vi "Pulse Pattern.vi"(10 "Selector":T1) -> (2 "Array":u16[](array[numeric]))   [LabVIEW 2026]
uses:
  SideSelector.ctl
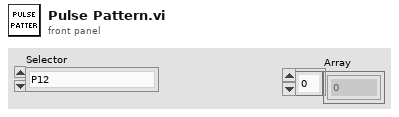
[diagram p1: front panel]
types:
  T1 = typedef "SideSelector.ctl" = enum16{"P12", "P1", "P2"}
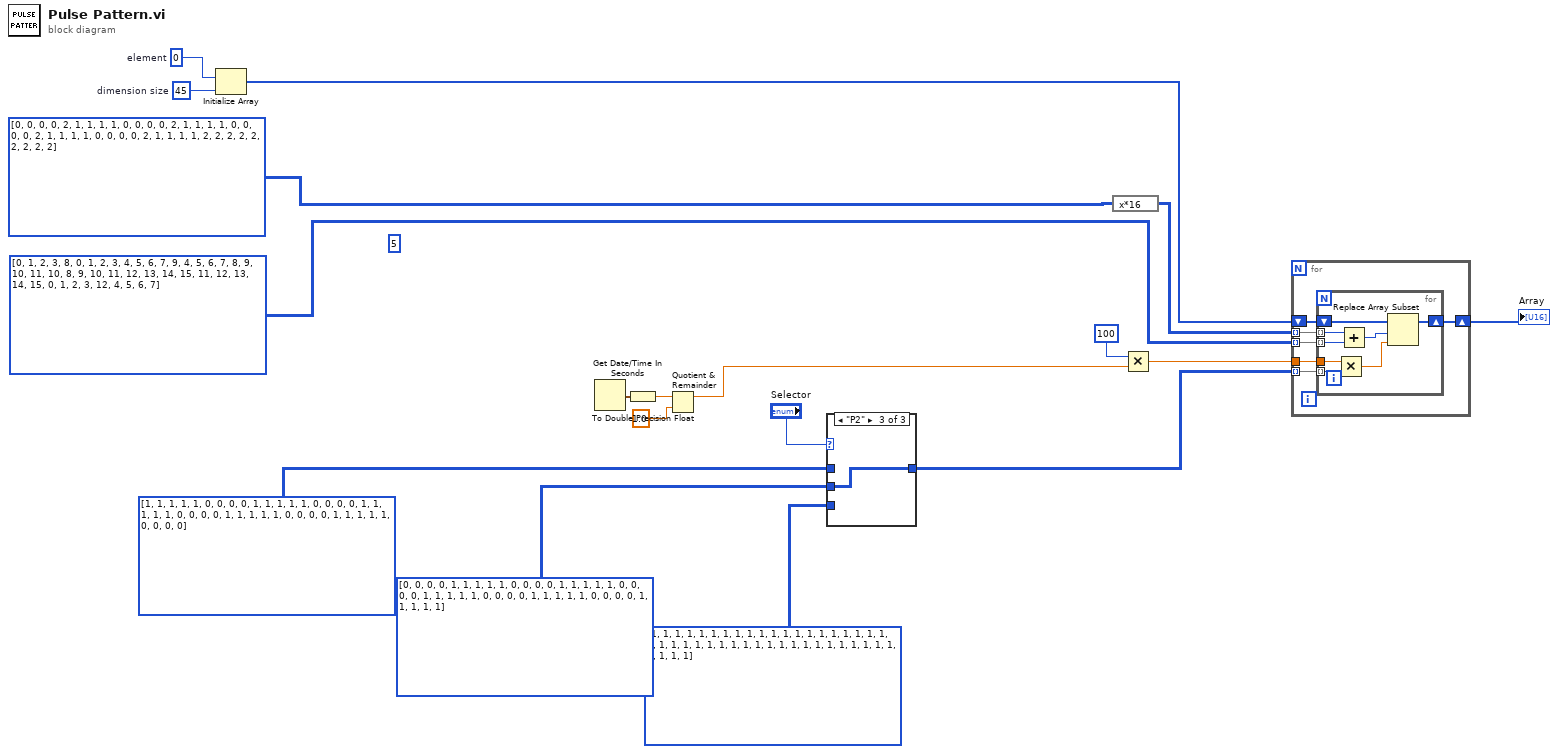
[diagram p0: block diagram]
diagram:
  (unwired) 5
  w17 = u16 0  # element
  w18 = 45  # dimension size
  n1 = Initialize Array(w17, w18) -> (w16:u16[])
  n2 = Get Date/Time In Seconds() -> (seconds since 1Jan1904=w13:timestamp)
  n3 = To Double Precision Float(number=w13) -> (double precision float=w12:dbl)
  n4 = Quotient & Remainder(x=w12, y=1.0) -> (x-y*floor(x/y)=w2:dbl)  [unwired: 1 out]
  n5 = case shown="\"P2\"" "Selector" {
    tunnel: [w19 w20 w21] -> w6
    tunnel: i32[][] [[1, 1, 1, 1, 1, 0, 0, 0, 0], [1, 1, 1, 1, 1, 0, 0, 0, 0], [1, 1, 1, 1, 1, 0, 0, 0, 0], [1, 1, 1, 1, 1, 0, 0, 0, 0], [1, 1, 1, 1, 1, 0, 0, 0, 0]] -> [_ w20 _]
    tunnel: i32[][] [[1, 1, 1, 1, 1, 1, 1, 1, 1], [1, 1, 1, 1, 1, 1, 1, 1, 1], [1, 1, 1, 1, 1, 1, 1, 1, 1], [1, 1, 1, 1, 1, 1, 1, 1, 1], [1, 1, 1, 1, 1, 1, 1, 1, 1]] -> [w19 _ _]
    tunnel: i32[][] [[0, 0, 0, 0, 1, 1, 1, 1, 1], [0, 0, 0, 0, 1, 1, 1, 1, 1], [0, 0, 0, 0, 1, 1, 1, 1, 1], [0, 0, 0, 0, 1, 1, 1, 1, 1], [0, 0, 0, 0, 1, 1, 1, 1, 1]] -> [_ _ w21]
    frame "P12" {
    }
    frame "P1" {
    }
    frame "P2" {
    }
  }
  n6 = expression code="x*16"(i32[][] [[0, 0, 0, 0, 2, 1, 1, 1, 1], [0, 0, 0, 0, 2, 1, 1, 1, 1], [0, 0, 0, 0, 2, 1, 1, 1, 1], [0, 0, 0, 0, 2, 1, 1, 1, 1], [2, 2, 2, 2, 2, 2, 2, 2, 2]]) -> (w8:i32[][])
  n7 = Multiply(x=100, y=w2) -> (x*y=w10:dbl)
  n8 = for {
    shift-right: [w26] -> w7
    shift-left: w16 -> [w27]
    tunnel: w10 -> [w25]
    tunnel: w8 -> [w24] mode=indexing
    tunnel: i32[][] [[0, 1, 2, 3, 8, 0, 1, 2, 3], [4, 5, 6, 7, 9, 4, 5, 6, 7], [8, 9, 10, 11, 10, 8, 9, 10, 11], [12, 13, 14, 15, 11, 12, 13, 14, 15], [0, 1, 2, 3, 12, 4, 5, 6, 7]] -> [w23] mode=indexing
    tunnel: w6 -> [w22] mode=indexing
    n9 = for {
      shift-right: [w34] -> w26
      shift-left: w27 -> [w35]
      tunnel: w25 -> [w33]
      tunnel: w24 -> [w32] mode=indexing
      tunnel: w23 -> [w31] mode=indexing
      tunnel: w22 -> [w28] mode=indexing
      n10 = Multiply(x=w33, y=w28) -> (x*y=w29:dbl)
      n11 = Add(x=w32, y=w31) -> (x+y=w30:i32)
      n12 = Replace Array Subset(array=w35, new element=w29, index=w30) -> (w34:u16[])
    }
  }
  "Array" <- w7
